vi "test Get Chamber Status-Test Status.vi"(8 "error in (no error)":errorcluster, 11 "TestCase in":refnum<class "Get Chamber Status.lvclass">) -> (0 "error out":errorcluster, 3 "TestCase out":refnum<class "Get Chamber Status.lvclass">)   [LabVIEW 2018, in "Get Chamber Status.lvclass"]
uses:
  Get Chamber Status.lvclass
  Libraries/Thermal Chamber Response Simulator/Thermal Chamber Response Simulator.lvlib
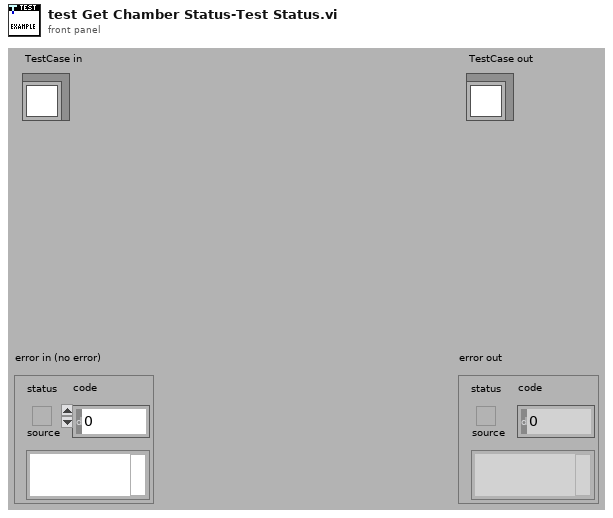
[diagram p1: front panel]
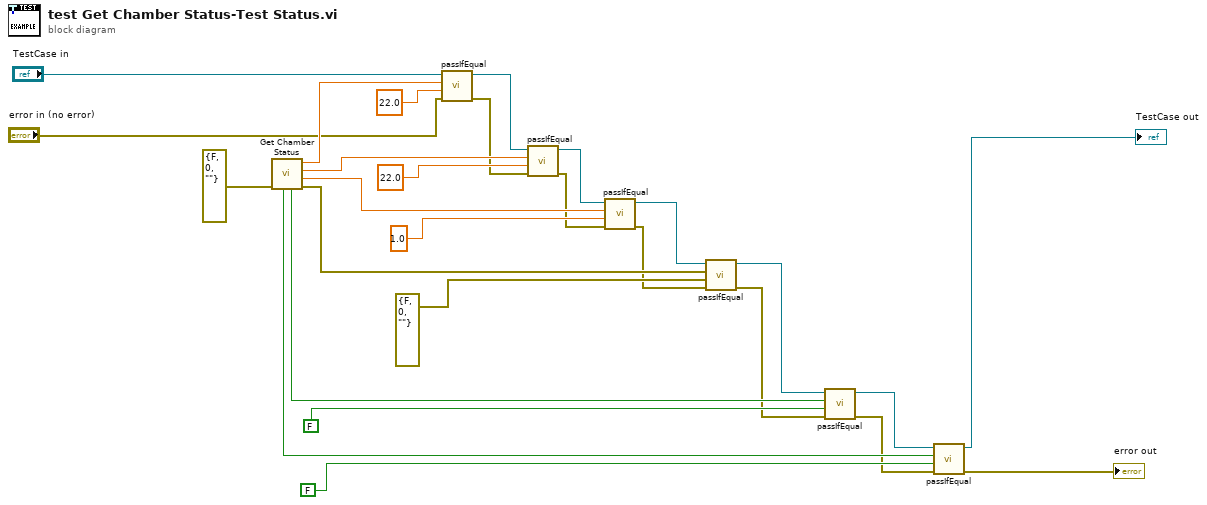
[diagram p0: block diagram]
diagram:
  n1 = call "Get Chamber Status.vi"("error in (no error)"=errorcluster {"status"=FALSE, "code"=0, "source"=""}) -> ("error out"=w21:errorcluster, "Ramp Rate (deg C / second)"=w22:dbl, "Temperature Set Point (deg C)"=w23:dbl, "Actual Temperature"=w27:dbl, "Application Exit"=w19:bool, "Heater State"=w18:bool)  [unwired: 5 in]
  n2 = call-dynamic "passIfEqual.vi"("error in (no error)"="error in (no error)", "y"=22.0 ("Actual Temperature"), "x"=w27, "TestCase in"="TestCase in") -> ("error out"=w3:errorcluster, "TestCase out"=w14:refnum<class "Get Chamber Status.lvclass">)  [unwired: 6 in]
  n3 = call-dynamic "passIfEqual.vi"("error in (no error)"=w3, "y"=22.0 ("Actual Temperature"), "x"=w23, "TestCase in"=w14) -> ("error out"=w4:errorcluster, "TestCase out"=w13:refnum<class "Get Chamber Status.lvclass">)  [unwired: 6 in]
  n4 = call-dynamic "passIfEqual.vi"("error in (no error)"=w4, "y"=1.0 ("Actual Temperature"), "x"=w22, "TestCase in"=w13) -> ("error out"=w5:errorcluster, "TestCase out"=w12:refnum<class "Get Chamber Status.lvclass">)  [unwired: 6 in]
  n5 = call-dynamic "passIfEqual.vi"("error in (no error)"=w5, "y"=errorcluster {"status"=FALSE, "code"=0, "source"=""} ("error out"), "x"=w21, "TestCase in"=w12) -> ("error out"=w6:errorcluster, "TestCase out"=w11:refnum<class "Get Chamber Status.lvclass">)  [unwired: 6 in]
  n6 = call-dynamic "passIfEqual.vi"("error in (no error)"=w6, "y"=FALSE ("Application Exit"), "x"=w19, "TestCase in"=w11) -> ("error out"=w7:errorcluster, "TestCase out"=w10:refnum<class "Get Chamber Status.lvclass">)  [unwired: 6 in]
  n7 = call-dynamic "passIfEqual.vi"("error in (no error)"=w7, "y"=FALSE ("Application Exit"), "x"=w18, "TestCase in"=w10) -> ("error out"=→"error out":errorcluster, "TestCase out"=→"TestCase out":refnum<class "Get Chamber Status.lvclass">)  [unwired: 6 in]
